vi "Excel Driver.vi"(0 "Option":T7, 2 "File name":string, 5 "Workbook":T5, 7 "Hyperlink":T3, 9 "Write/Read Cell":T6={"Cell Range"="", "Data 2D"=[], "Select Sheet"="", "1 Data"="", "Data 1D"=[], "Font col"=0, "Bold"=TRUE, "Font Size"=18, "Inside lines"=FALSE}, 11 "error in":errorcluster, 12 "Cell Parameters":T1={"Cell Range"="", "Horizontal Alignment"=enum."xlcenter", "Vertical Alignment"=enum."xlbottom"}, 14 "Write/Read Cell Numeric":T4 {"Data 1D" format="%.2f"; "Data 2D" format="%.2f"; "1 Data" format="%.2f"}) -> (1 "Last row used:":u64, 3 "Last column used:":u64, 4 "Data":string[][](array[string]), 6 "Single data From XL":string, 10 "Sheet Name":string[](array[string]), 15 "error out":errorcluster)   [LabVIEW 2017]
uses:
  controls/Excel.ctl
  controls/read.write.ctl
panel:
  in  "Print":T2
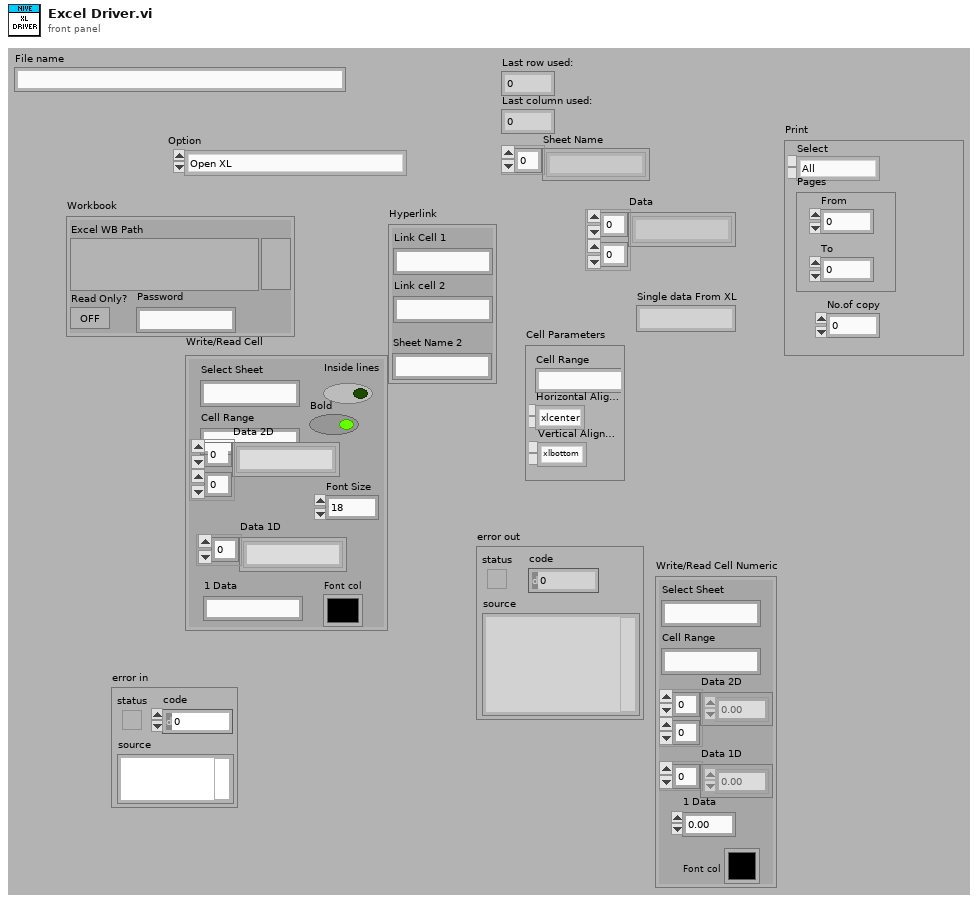
[diagram p1: front panel]
types:
  T1 = cluster{"Cell Range":string, "Horizontal Alignment":enum16{"xlnone", "xlgeneral", "xlleft", "xlcenter", "xlright"}, "Vertical Alignment":enum16{"xlnone", "xltop", "xlcentet", "xlbottom"}}
  T2 = cluster{"Select":enum16{"All", "From&To"}, "Pages":cluster{"From":u8, "To":u8}, "No.of copy":u8}
  T3 = cluster{"Link cell 2":string, "Link Cell 1":string, "Sheet Name 2":string}
  T4 = cluster{"Cell Range":string, "Select Sheet":string, "1 Data":dbl, "Data 2D":dbl[][], "Data 1D":dbl[], "Font col":u32}
  T5 = cluster{"Excel WB Path":path, "Read Only?":bool, "Password":string}
  T6 = typedef "read.write.ctl" = cluster{"Cell Range":string, "Data 2D":string[][], "Select Sheet":string, "1 Data":string, "Data 1D":string[], "Font col":u32, "Bold":bool, "Font Size":i32, "Inside lines":bool}
  T7 = typedef "Excel.ctl" = enum16{"Open XL", "Create Hyperlink within Sheet", "Create Hyperlink between Sheets", "Hyperlink Folders", "Read Sheet names", "Print", "Print Preview", "print", "Open WB", "Copy Sheets", "Copy sheet to sheet", "Add Sheets", "Select Sheet", "Paste CLPBRD", "Read 1 Cell", "Read 2D", "Write 1 Cell", "Write 1 Cell No", "Write 2D String", "Write 2D Double", "Write 1D String", "Write 1D Double", "Merge Cells", "Borders", "Save", "Save As PDF", "Get Last Row Column Number", "Close Sheet", "Delete Sheet", "Close WB", "Close XL"}
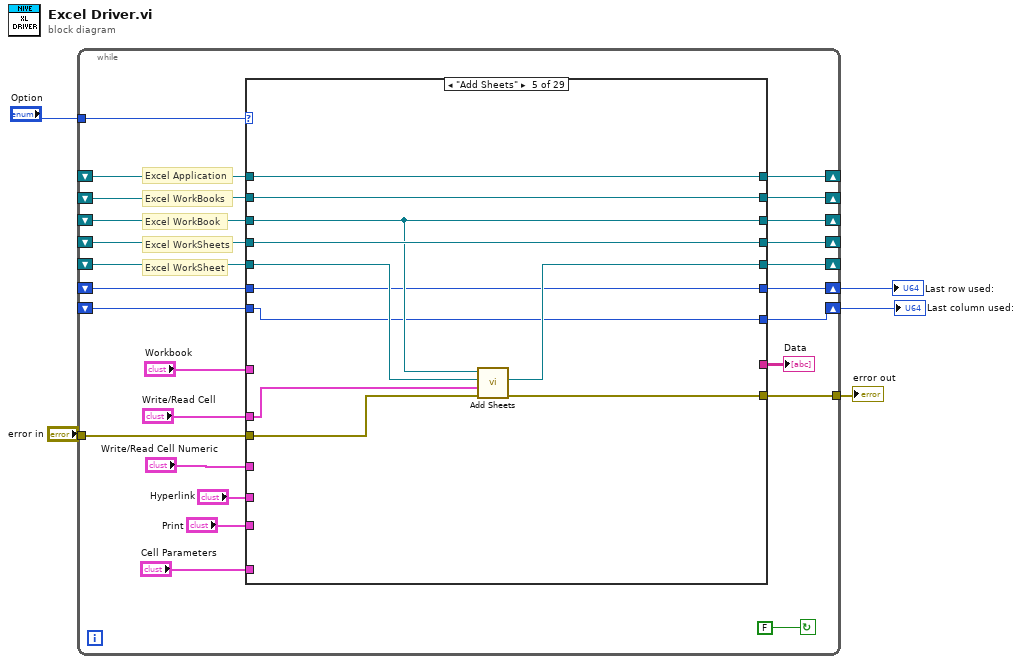
[diagram p0: block diagram]
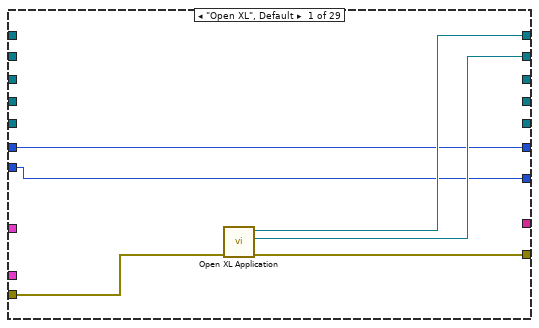
[diagram p2: hidden frame]
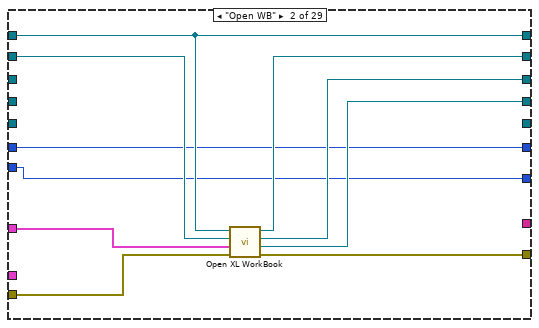
[diagram p3: hidden frame]
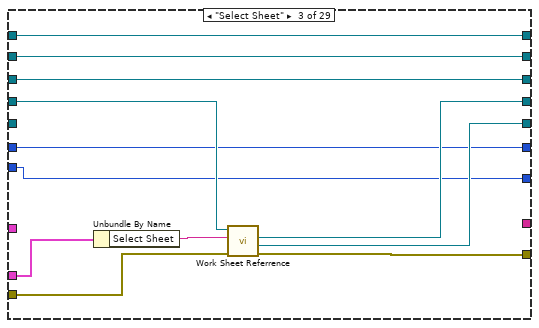
[diagram p4: hidden frame]
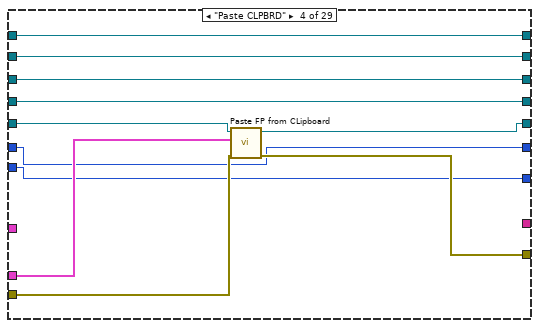
[diagram p5: hidden frame]
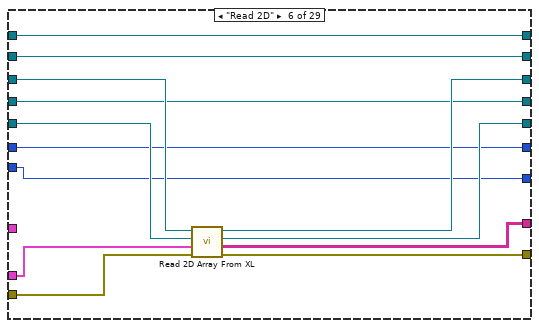
[diagram p6: hidden frame]
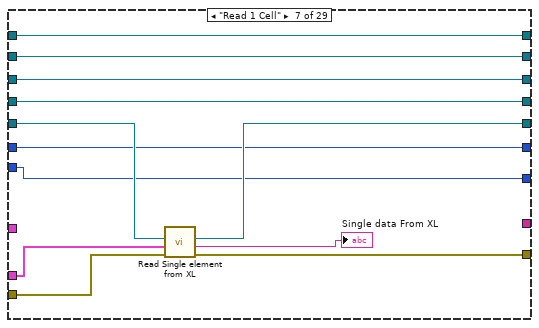
[diagram p7: hidden frame]
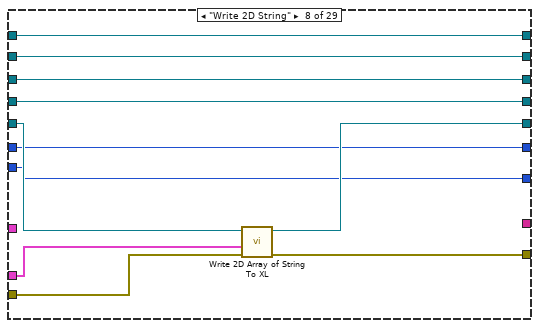
[diagram p8: hidden frame]
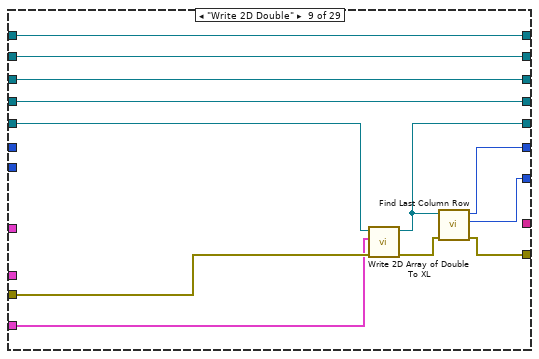
[diagram p9: hidden frame]
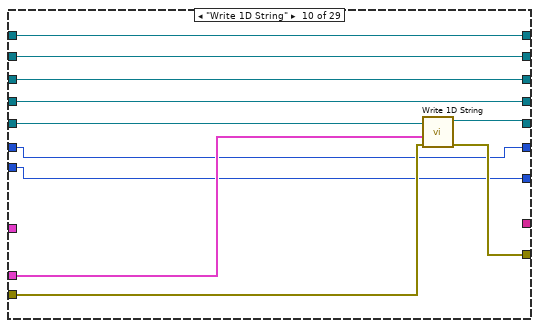
[diagram p10: hidden frame]
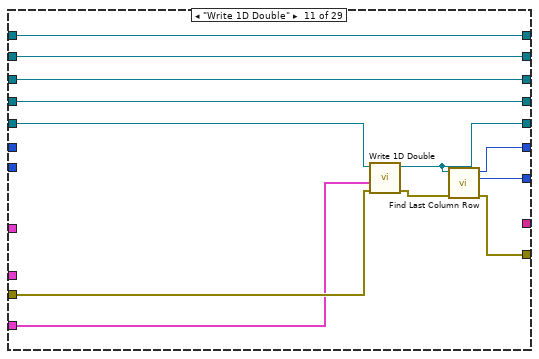
[diagram p11: hidden frame]
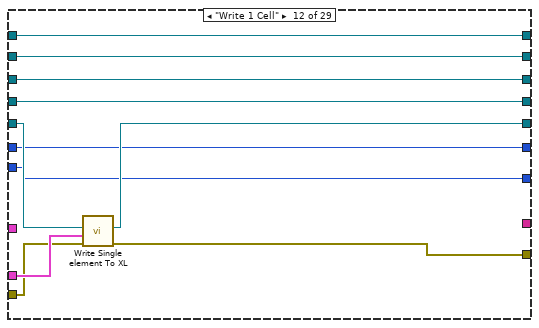
[diagram p12: hidden frame]
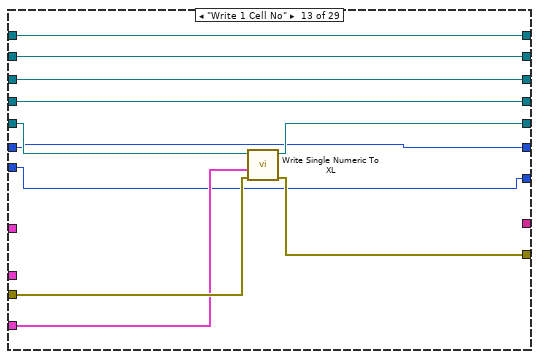
[diagram p13: hidden frame]
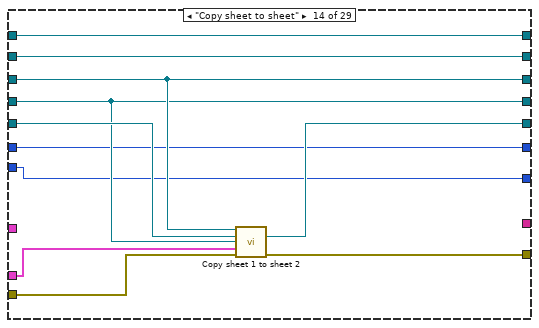
[diagram p14: hidden frame]
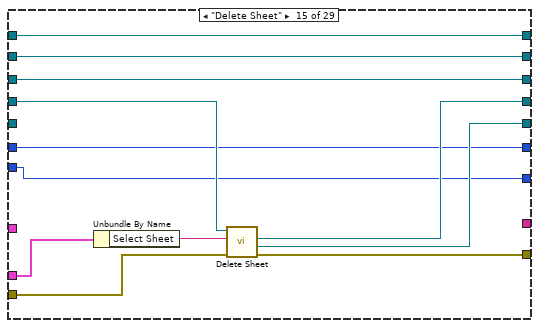
[diagram p15: hidden frame]
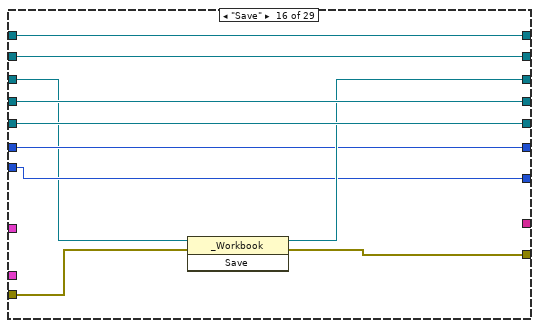
[diagram p16: hidden frame]
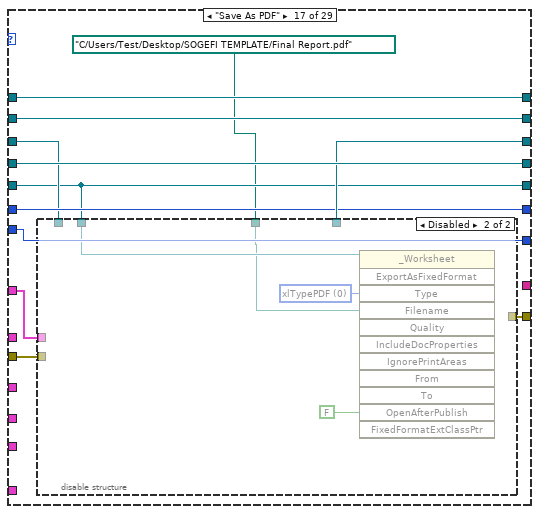
[diagram p17: hidden frame]
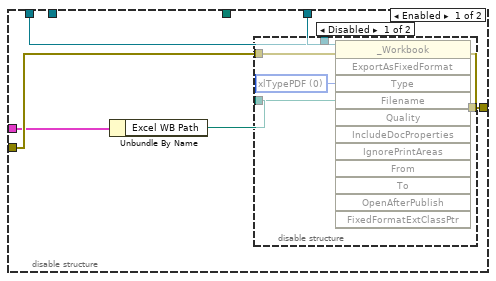
[diagram p18: hidden frame]
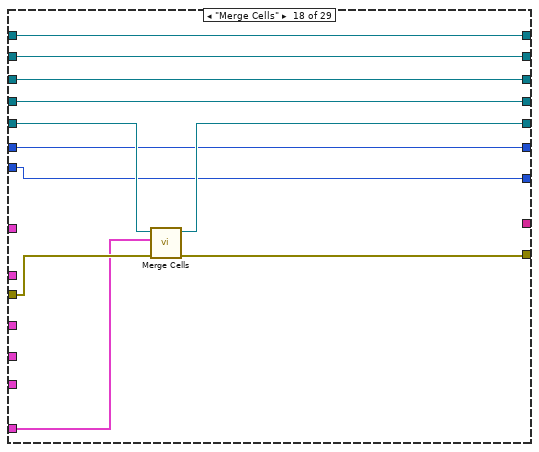
[diagram p20: hidden frame]
diagram:
  n1 = while {
    shift-right: [w28] -> _
    shift-left: _ -> [w25]
    shift-right: [w27] -> _
    shift-left: _ -> [w24]
    shift-right: [w23] -> _
    shift-left: _ -> [w13]
    shift-right: [w22] -> _
    shift-left: _ -> [w21]
    tunnel: "Option" -> [w29]
    tunnel: "error in" -> [w26]
    tunnel: [w10] -> w5
    shift-right: [w11] -> _
    shift-left: _ -> [w20]
    shift-right: [w9] -> w2
    shift-left: _ -> [w7]
    shift-right: [w8] -> w1
    shift-left: _ -> [w6]
    stop <- FALSE continue-if-true
    # "Excel WorkSheet"
    # "Excel WorkSheets"
    # "Excel WorkBook"
    # "Excel WorkBooks"
    # "Excel Application"
    n2 = case shown="\"Add Sheets\"" w29 {
      tunnel: [w36 w43 w54 w65 w80 w90 w105 w114 w126 w139 w151 w162 w173 w184 w192 w206 w218 w240 w248 w262 w280 w296 w300 w320 w337 w348 w357 w368 _] -> w28
      tunnel: [w35 w40 w53 w64 w79 w89 w104 w113 w125 w138 w150 w161 w172 w183 w191 w200 w213 w239 w249 w261 w279 w295 w301 w319 w336 w347 w356 w364 _] -> w27
      tunnel: w26 -> [w33 w46 w58 w68 w74 w93 w100 w116 w128 w132 w146 w155 w169 w178 w196 w203 w216 w245 w253 w264 w282 w290 w306 w322 w339 w344 w353 w363 w375]
      tunnel: [w34 w45 w57 w66 w73 w92 w99 w115 w120 w133 w140 w154 w168 w179 w195 w202 w215 w244 w252 w268 w286 w290 w305 w321 w338 w343 w352 w361 w374] -> w10
      tunnel: w25 -> [_ w43 w54 w65 w80 w90 w105 w114 w126 w139 w151 w162 w173 w184 w192 w206 w218 w240 w248 w266 w284 w296 w300 w320 w337 w348 w357 w360 w373]
      tunnel: w24 -> [_ w44 w53 w64 w79 w89 w104 w113 w125 w138 w150 w161 w172 w183 w191 w200 w213 w239 w249 w261 w279 w295 w301 w319 w336 w347 w356 w364 _]
      tunnel: [_ w42 w50 w63 w77 w88 w103 w112 w124 w137 w149 w160 w171 w182 w188 w201 w214 w238 w250 w260 w278 w294 w302 w317 w334 w346 w355 _ _] -> w23
      tunnel: [_ w41 w56 w62 w78 w85 w102 w111 w123 w136 w148 w159 w170 w176 w194 w205 w217 w237 w251 w259 w277 w292 w303 w314 w328 w345 w354 _ _] -> w22
      tunnel: [_ _ w55 w67 w75 w87 w96 w110 w119 w134 w144 w156 w167 w180 w193 w204 w209 w242 w255 w269 w287 w293 w304 w313 w331 w342 _ _ _] -> w11
      tunnel: w21 -> [_ _ w49 w62 w78 w85 w102 w111 w123 w136 w148 w159 w170 w176 w187 w205 w217 w237 w251 w259 w277 w292 w303 w314 w328 w345 w354 w367 _]
      tunnel: w20 -> [_ _ _ w69 w76 w86 w97 w108 w127 w135 w147 w157 w166 w181 _ w204 w209 w243 w256 w267 w285 w297 w304 w313 w331 w342 w351 _ _]
      tunnel: [_ _ _ _ _ w84 _ _ _ _ _ _ _ _ _ _ _ _ _ _ _ _ _ _ _ _ _ _ _] -> w19
      tunnel: "Write/Read Cell" -> [_ _ w52 w61 w72 w83 w101 w109 _ w131 _ w158 _ w177 w190 _ _ _ w254 _ _ _ _ w318 w335 _ _ _ _]
      tunnel: "Workbook" -> [_ w39 _ _ _ _ _ _ _ _ _ _ _ _ _ _ w207 _ _ _ _ _ _ w316 w333 _ _ w365 _]
      tunnel: "Write/Read Cell Numeric" -> [_ _ _ _ _ _ _ _ w122 _ w145 _ w165 _ _ _ _ _ _ _ _ _ _ _ _ _ _ _ _]
      tunnel: "Hyperlink" -> [_ _ _ _ _ _ _ _ _ _ _ _ _ _ _ _ _ _ _ _ _ _ _ w312 w330 _ _ _ _]
      tunnel: "Print" -> [_ _ _ _ _ _ _ _ _ _ _ _ _ _ _ _ _ _ _ _ _ _ _ _ _ _ _ _ _]
      tunnel: "Cell Parameters" -> [_ _ _ _ _ _ _ _ _ _ _ _ _ _ _ _ _ w241 _ _ _ _ _ _ _ _ _ _ _]
      tunnel: w13 -> [_ _ w50 w63 w77 w91 w103 w112 w124 w137 w149 w160 w171 w182 w188 w197 w210 w238 w250 w260 w278 w294 w302 w317 w334 w346 w355 w366 _]
      tunnel: [w32 w38 w48 w60 w71 w82 w95 w107 w118 w130 w143 w153 w164 w175 w186 w199 w212 w236 w247 w258 w276 w289 w299 w308 w324 w341 w350 w359 w372] -> w9
      tunnel: [w31 w37 w47 w59 w70 w81 w94 w106 w117 w129 w142 w152 w163 w174 w185 w198 w211 w235 w246 w257 w272 w288 w298 w307 w323 w340 w349 w358 w371] -> w8
      tunnel: w7 -> [w32 w38 w48 w60 w71 w82 w95 w107 _ w130 _ w153 w164 w175 w186 w199 w212 w236 w247 w258 w276 w289 _ w308 w324 w341 w350 w359 w372]
      tunnel: w6 -> [w31 w37 w47 w59 w70 w81 w94 w106 _ w129 _ w152 w163 w174 w185 w198 w211 w235 w246 w257 w272 w288 _ w307 w323 w340 w349 w358 w371]
      frame "Open XL", Default {
        n3 = call "Open XL Application.vi"("error in"=w33) -> ("error out"=w34:errorcluster, "Excel.Workbooks"=w35:refnum<k7>, "Excel._Application"=w36:refnum<k7>)  [unwired: 8 out]
      }
      frame "Open WB" {
        n4 = call "Open XL WorkBook.vi"("error in"=w46, "Workbook"=w39, "Workbooks"=w44, "Excel._Application"=w43) -> ("error out"=w45:errorcluster, "Sheets"=w41:refnum<k7>, "Excel._Workbook"=w42:refnum<k7>, "Excel.Workbooks"=w40:refnum<k7>)  [unwired: 4 out]
      }
      frame "Select Sheet" {
        n5 = Unbundle By Name(w52) -> ("Select Sheet"=w51:string)
        n6 = call "Work Sheet Referrence.vi"("error in"=w58, "Sheet Name"=w51, "Worksheets 2"=w49) -> ("error out"=w57:errorcluster, "Work Sheet"=w55:refnum<k7>, "Worksheets"=w56:refnum<k7>)  [unwired: 6 out]
      }
      frame "Paste CLPBRD" {
        n7 = call "Paste FP from CLipboard.vi"("error in"=w68, "Write/Read Cell"=w61, "Work Sheet 2"=w69) -> ("error out"=w66:errorcluster, "Work Sheet"=w67:refnum<k7>)  [unwired: 7 in]
      }
      frame "Add Sheets" {
        n8 = call "Add Sheets.vi"("error in"=w74, "Write/Read Cell"=w72, "Work Sheet"=w76, "Excel._Workbook"=w77) -> ("error out"=w73:errorcluster, "Work Sheet"=w75:refnum<k7>)  [unwired: 6 out]
      }
      frame "Read 2D" {
        n9 = call "Read 2D Array From XL.vi"("error in"=w93, "Write/Read Cell"=w83, "Work Sheet"=w86, "Excel._Workbook"=w91) -> ("error out"=w92:errorcluster, "Data From Cells"=w84:string[][], "Work Sheet"=w87:refnum<k7>, "Excel._Workbook"=w88:refnum<k7>)  [unwired: 4 out]
      }
      frame "Read 1 Cell" {
        n10 = call "Read Single element from XL.vi"("error in"=w100, "Write/Read Cell"=w101, "Work Sheet"=w97) -> ("error out"=w99:errorcluster, "data From XL"=→"Single data From XL":string, "Work Sheet"=w96:refnum<k7>)  [unwired: 6 out]
      }
      frame "Write 2D String" {
        n11 = call "Write 2D Array of String To XL.vi"("error in"=w116, "Write/Read Cell"=w109, "Work Sheet"=w108) -> ("error out"=w115:errorcluster, "Work Sheet"=w110:refnum<k7>)  [unwired: 1 in, 6 out]
      }
      frame "Write 2D Double" {
        n12 = call "Write 2D Array of Double To XL.vi"("error in"=w128, "Write/Read Cell Numeric"=w122, "Work Sheet"=w127) -> ("error out"=w121:errorcluster, "Work Sheet"=w119:refnum<k7>)  [unwired: 1 in, 6 out]
        n13 = call "Find Last Column Row.vi"("error in"=w121, "Excel._Worksheet"=w119) -> ("error out"=w120:errorcluster, "Last column used:"=w117:u64, "Last row used:"=w118:u64)  [unwired: 7 out]
      }
      frame "Write 1D String" {
        n14 = call "Write 1D String.vi"("error in"=w132, "Write/Read Cell"=w131, "Work Sheet 2"=w135) -> ("error out"=w133:errorcluster, "Work Sheet"=w134:refnum<k7>)  [unwired: 7 out]
      }
      frame "Write 1D Double" {
        n15 = call "Write 1D Double.vi"("error in"=w146, "Write/Read Cell Numeric"=w145, "Work Sheet 2"=w147) -> ("error out"=w141:errorcluster, "Work Sheet"=w144:refnum<k7>)  [unwired: 7 out]
        n16 = call "Find Last Column Row.vi"("error in"=w141, "Excel._Worksheet"=w144) -> ("error out"=w140:errorcluster, "Last column used:"=w142:u64, "Last row used:"=w143:u64)  [unwired: 7 out]
      }
      frame "Write 1 Cell" {
        n17 = call "Write Single element To XL.vi"("error in"=w155, "Write/Read Cell"=w158, "Work Sheet"=w157) -> ("error out"=w154:errorcluster, "Work Sheet"=w156:refnum<k7>)  [unwired: 7 out]
      }
      frame "Write 1 Cell No" {
        n18 = call "Write Single Numeric To XL.vi"("error in"=w169, "Write/Read Cell Numeric"=w165, "Work Sheet 2"=w166) -> ("error out"=w168:errorcluster, "Work Sheet"=w167:refnum<k7>)  [unwired: 7 out]
      }
      frame "Copy sheet to sheet" {
        n19 = call "Copy sheet 1 to sheet 2.vi"("Excel._Workbook"=w182, "Work Sheet"=w181, "WorkSheets"=w176, "Write/Read Cell"=w177, "error in"=w178) -> ("Work Sheet"=w180:refnum<k7>, "error out"=w179:errorcluster)  [unwired: 9 out]
      }
      frame "Delete Sheet" {
        n20 = Unbundle By Name(w190) -> ("Select Sheet"=w189:string)
        n21 = call "Delete Sheet.vi"("error in"=w196, "Sheet Name"=w189, "Worksheets 2"=w187) -> ("error out"=w195:errorcluster, "Work Sheet"=w193:refnum<k7>, "Worksheets"=w194:refnum<k7>)  [unwired: 6 out]
      }
      frame "Save" {
        n22 = invoke class="_Workbook" method="Save"(reference=w197, error in=w203) -> (reference out=w201:refnum<k7>, error out=w202:errorcluster)  [unwired: 1 in, 1 out]
      }
      frame "Save As PDF" {
        n23 = disable-structure shown="Disabled" {
          disable-tunnel: w216 -> [w224 _]
          disable-tunnel: [w221 _] -> w215
          disable-tunnel: [w223 _] -> w214
          disable-tunnel: w210 -> [w222 _]
          disable-tunnel: w209 -> [_ w232]
          disable-tunnel: path "C:/Users/Test/Desktop/SOGEFI TEMPLATE/Final Report.pdf" -> [_ w231]
          disable-tunnel: w207 -> [w220 _]
          frame Enabled {
            n24 = Unbundle By Name(w220) -> ("Excel WB Path"=w219:path)
            n25 = disable-structure shown="Disabled" {
              disable-tunnel: w224 -> [w230 _]
              disable-tunnel: [w229 _] -> w223
              disable-tunnel: w222 -> [w228 _]
              disable-tunnel: [w226 _] -> w221
              disable-tunnel: w219 -> [w225 _]
              frame Disabled {
                w227 = 0 items=["xlTypePDF", "xlTypeXPS"] ("Type")
                n26 = invoke class="_Workbook" method="ExportAsFixedFormat"(reference=w228, error in=w230, "Type"=w227, "Filename"=w225) -> (reference out=w229:refnum<k7>, error out=w226:errorcluster)  [unwired: 8 in, 10 out]
              }
              frame Enabled {
              }
            }
          }
          frame Disabled {
            w234 = 0 items=["xlTypePDF", "xlTypeXPS"] ("Type")
            n27 = invoke class="_Worksheet" method="ExportAsFixedFormat"(reference=w232, "Type"=w234, "Filename"=w231, "OpenAfterPublish"=FALSE) -> ()  [unwired: 8 in, 12 out]
          }
        }
      }
      frame "Merge Cells" {
        n28 = call "Merge Cells.vi"("error in"=w245, "Cell Parameters"=w241, "_Worksheet"=w243) -> ("error out"=w244:errorcluster, "_Worksheet"=w242:refnum<k7>)  [unwired: 7 out]
      }
      frame "Borders" {
        n29 = call "Borders.vi"("error in"=w253, "Write/Read Cell"=w254, "_Worksheet 2"=w256) -> ("error out"=w252:errorcluster, "_Worksheet"=w255:refnum<k7>)  [unwired: 7 in]
      }
      frame "Print Preview" {
        n30 = property class="_Application"(reference=w266, error in=w264, "Visible"=TRUE) -> (reference out=w262:refnum<k7>, error out=w263:errorcluster)
        n31 = invoke class="_Worksheet" method="PrintPreview"(reference=w267, error in=w263) -> (reference out=w269:refnum<k7>, error out=w268:errorcluster)  [unwired: 2 in, 2 out]
      }
      frame "Print" {
        n32 = property class="_Application"(reference=w284, error in=w282, "Visible"=FALSE) -> (reference out=w280:refnum<k7>, error out=w281:errorcluster)
        n33 = To Variant(anything="File name") -> (Variant=w273:variant)
        n34 = invoke class="_Worksheet" method="PrintOut"(reference=w285, error in=w281, "From"=1, "To"=2, "ActivePrinter"="Microsoft Print to PDF", "PrToFileName"=w273) -> (reference out=w287:refnum<k7>, error out=w286:errorcluster)  [unwired: 6 in, 10 out]
      }
      frame "Read Sheet names" {
        n35 = call "Sheet Names.vi"("Excel._Worksheet"=w297, "Worksheets"=w292) -> ("Sheet Name"=→"Sheet Name":string[], "Excel._Worksheet"=w293:refnum<k7>)  [unwired: 8 out]
      }
      frame "Get Last Row Column Number" {
        n36 = call "Find Last Column Row.vi"("error in"=w306, "Excel._Worksheet"=w304) -> ("error out"=w305:errorcluster, "Last column used:"=w298:u64, "Last row used:"=w299:u64)  [unwired: 7 out]
      }
      frame "Create Hyperlink within Sheet" {
        # "This case is for create the hyperlink between the two cells in the sheet itself."
        n37 = Unbundle By Name(w316) -> ("Excel WB Path"=w315:path)
        n38 = Unbundle By Name(w312) -> ("Link Cell 1"=w310:string, "Link cell 2"=w309:string)
        n39 = Unbundle By Name(w318) -> ("Select Sheet"=w311:string)
        n40 = call "Create Hyperlink.vi"("Work Sheet"=w313, "File Path"=w315, "Sheet Name"=w311, "Link Cell 1"=w310, "Link Cell 2"=w309, "error in"=w322) -> ("error out"=w321:errorcluster)  [unwired: 9 out]
      }
      frame "Create Hyperlink between Sheets" {
        # "This case is for create the hyperlink between the two Sheets in One XL file"
        n41 = Unbundle By Name(w333) -> ("Excel WB Path"=w332:path)
        n42 = Unbundle By Name(w330) -> ("Sheet Name 2"=w325:string, "Link Cell 1"=w329:string, "Link cell 2"=w327:string)
        n43 = Unbundle By Name(w335) -> ("Select Sheet"=w326:string)
        n44 = call "Create Hyperlink between 2 sheets.vi"("Work Sheet"=w331, "Sheet Name 2"=w325, "Sheet Name 1"=w326, "Link Cell 1"=w329, "Link Cell 2"=w327, "error in"=w339, "File Path"=w332, "Worksheets"=w328) -> ("error out"=w338:errorcluster)  [unwired: 4 in, 7 out]
      }
      frame "Hyperlink Folders" {
        n45 = call "Create Hyperlink Folders.vi"("Work Sheet"=w342, "error in"=w344) -> ("error out"=w343:errorcluster)  [unwired: 17 out]
      }
      frame "Close Sheet" {
        n46 = Close Reference(reference=w351, error in (no error)=w353) -> (error out=w352:errorcluster)
      }
      frame "Close WB" {
        n47 = stacked-sequence {
          tunnel: w367 -> [w370]
          tunnel: w363 -> [w369]
          tunnel: [w369] -> w362
          frame #0 {
            n48 = Close Reference(reference=w370) -> ()  [unwired: 1 in, 1 out]
          }
        }
        n49 = call "Close XL WorkBook.vi"("error in"=w362, "Workbook"=w365, "Excel._Workbook"=w366, "Excel._Application"=w360) -> ("error out"=w361:errorcluster, "Excel._Application"=w368:refnum<k7>)  [unwired: 6 out]
      }
      frame "Close XL" {
        n50 = call "Close XL Application.vi"("error in"=w375, "Excel._Application"=w373) -> ("error out"=w374:errorcluster)  [unwired: 9 out]
      }
    }
    "Data" <- w19
  }
  "error out" <- w5
  "Last row used:" <- w2
  "Last column used:" <- w1
